vi "_MatchRefMasses.vi"(2 "Cal/Res Table":dbl[][](array[numeric]) format="%.2f", 3 "MassReference":cluster{"Mass":dbl, "Use":bool}[](array[cluster])) -> (0 "Cal/Res Table Out":dbl[][](array[numeric]) format="%.2f")   [LabVIEW 2015]
uses:
  Type/_Log Command.ctl
panel:
  out "slope":dbl[](array[numeric])
  # "Ensure a calibration / resolution table contain all reference masses\nthat are in use and no others."
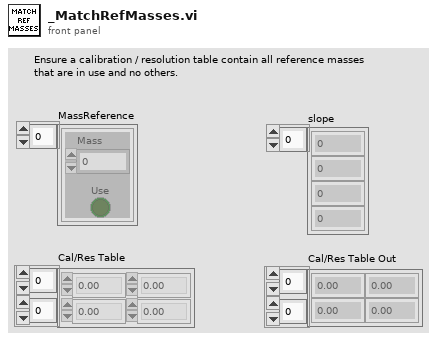
[diagram p1: front panel]
types:
  T1 = typedef "_Log Command.ctl" = enum16{"No Command", "Open", "Read", "Write", "Close", "Check Size"}
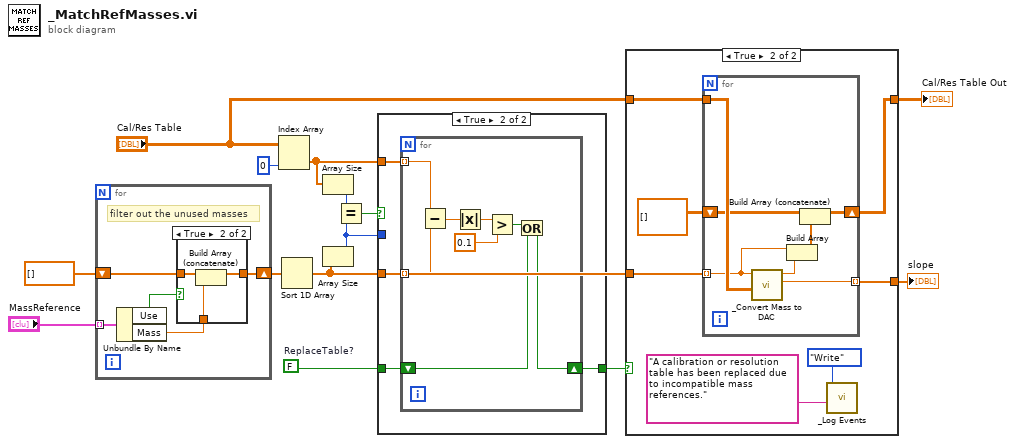
[diagram p0: block diagram]
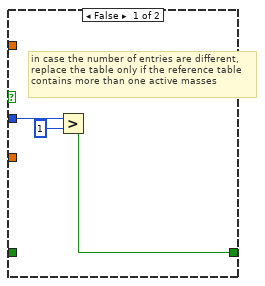
[diagram p3: hidden frame]
diagram:
  w14 = FALSE  # ReplaceTable?
  n1 = for {
    shift-right: [w16] -> w11
    shift-left: dbl[] [] -> [w17]
    tunnel: "MassReference" -> [w19] mode=indexing
    # "filter out the unused masses"
    n2 = Unbundle By Name(w19) -> ("Use"=w18:bool, "Mass"=w15:dbl)
    n3 = case shown="True" w18 {
      tunnel: w17 -> [w20 w23]
      tunnel: [w20 w22] -> w16
      tunnel: w15 -> [_ w21]
      frame False {
      }
      frame True {
        n4 = Build Array (concatenate)(w23, w21) -> (w22:dbl[])
      }
    }
  }
  n5 = Index Array(array="Cal/Res Table", index (col)=0 ("disabled index (col)")) -> (element=w6:dbl[])  [unwired: 1 in]
  n6 = Sort 1D Array(array=w11) -> (sorted array=w3:dbl[])
  n7 = Array Size(array=w6) -> (size(s)=w9:i32)
  n8 = Array Size(array=w3) -> (size(s)=w7:i32)
  n9 = Equal?(x=w9, y=w7) -> (x = y?=w8:bool)
  n10 = case shown="True" w8 {
    tunnel: w14 -> [_ w30]
    tunnel: w3 -> [_ w29]
    tunnel: [w24 w28] -> w5
    tunnel: w7 -> [w26 _]
    tunnel: w6 -> [_ w27]
    frame False {
      # "in case the number of entries are different,\nreplace the table only if the reference table\ncontains more than one active masses"
      n11 = Greater?(x=w26, y=1) -> (0:w24:bool)
    }
    frame True {
      n12 = for {
        shift-right: [w31] -> w28
        shift-left: w30 -> [w32]
        tunnel: w29 -> [w36] mode=indexing
        tunnel: w27 -> [w37] mode=indexing
        n13 = Subtract(x=w37, y=w36) -> (x-y=w38:dbl)
        n14 = Absolute Value(x=w38) -> (abs(x)=w35:dbl)
        n15 = Greater?(x=w35, y=0.1) -> (0:w33:bool)
        n16 = Or(x=w33, y=w32) -> (x .or. y?=w31:bool)
      }
    }
  }
  n17 = case shown="True" w5 {
    tunnel: "Cal/Res Table" -> [w39 w43]
    tunnel: w3 -> [_ w44]
    tunnel: [w39 w41] -> w2
    tunnel: [_ w40] -> w1
    frame False {
      # "no need to replace table"
    }
    frame True {
      n18 = for {
        tunnel: w44 -> [w52] mode=indexing
        tunnel: w43 -> [w53]
        shift-right: [w48] -> w41
        shift-left: dbl[][] [] -> [w50]
        tunnel: [w47] -> w40 mode=indexing
        n19 = call "_Convert Mass to DAC.vi"("Calibration Table"=w53, "Mass"=w52) -> ("Slope"=w47:dbl, "DAC Value"=w51:dbl)  [unwired: 2 in, 2 out]
        n20 = Build Array(w52, w51) -> (w49:dbl[])
        n21 = Build Array (concatenate)(w50, w49) -> (w48:dbl[][])
      }
      n22 = call "_Log Events.vi"("Event"="A calibration or resolution table has been replaced due to incompatible mass references.", "Log Command"=_Log_Command."Write") -> ()  [unwired: 6 in, 2 out]
    }
  }
  "Cal/Res Table Out" <- w2
  "slope" <- w1
